vi "Disable.vi"(8 "error in (no error)":errorcluster, 11 "NHRDCPower in":refnum<class "NHRDCPower.lvclass">) -> (0 "error out":errorcluster, 3 "NHRDCPower out":refnum<class "NHRDCPower.lvclass">)   [LabVIEW 2018, in "AcPwrPlugins.lvlib" / "NHRDCPower.lvclass"]
doc: "This VI disconnects the instruments output or input."
uses:
  NHRDCPower.lvclass
  <instrlib>/NHRDCPowerModule/NHRDCPowerModule/NHRDCPowerModule.lvlib
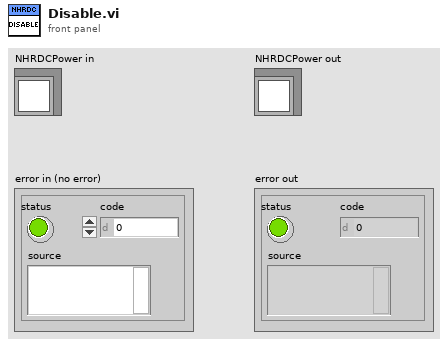
[diagram p1: front panel]
types:
  T1 = typedef "AcPwrPlugins.lvlib/NHRDCPower.lvclass/Device(s)Settings.ctl" = cluster{"Handle":string, "Name":string, "id query (Yes)":bool, "reset device (Yes)":bool, "Connected":bool, "Voltage Range (V)":dbl[], "Timing":cluster{"TimingOn":enum16{""}, "Hours":u32, "Minutes":u32, "Seconds":dbl, "CutoffVoltage":dbl}, "Initial Battery Detect Voltage (0)":sgl, "SafetySettings":cluster{"SetWatchDog":bool, "Voltage (V)":sgl, "Current (A)":sgl, "Power (W)":sgl, "Voltage Delay (s)":sgl, "Current Delay (s)":sgl, "Power Delay (s)":sgl}, "Options String":string, "Aperture Time (s)":sgl, "operating state (Off)":i32, "OutputSettings":cluster{"Voltage (V)":sgl, "Current (A)":sgl, "Resistance (Ohms)":sgl, "Power (W)":sgl, "Enable Voltage":bool, "Enable Current":bool, "Enable Resistance":bool, "Enable Power":bool, "Delay After (s)":sgl, "Wait Value (V, A, W)":sgl, "Enable Wait":bool, "Wait on Value":i32}[], "SlewRate":cluster{"Set Voltage Rate V/S":sgl, "Set Current Rate A/S":sgl, "Set Resistance Rate R/S":sgl, "Set Power Rate W/S":sgl}}[]
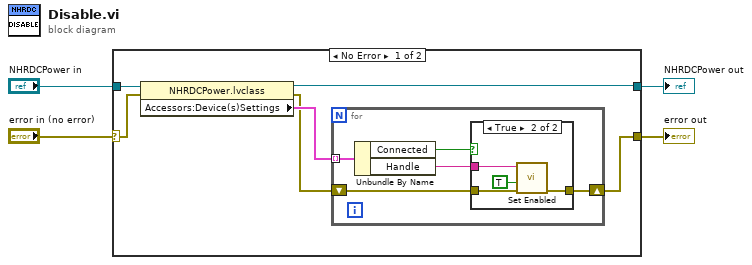
[diagram p0: block diagram]
diagram:
  n1 = case shown="No Error" "error in (no error)" {
    selector: "error in (no error)" -> [w9 w21]
    tunnel: [w5 w21] -> w1
    tunnel: [w6 w22] -> w2
    tunnel: "NHRDCPower in" -> [w10 w22]
    frame No Error {
      n2 = property class="NHRDCPower.lvclass"(reference=w10, error in=w9) -> (reference out=w6:refnum<class "NHRDCPower.lvclass">, error out=w7:errorcluster, "Accessors:Device(s)Settings"=w8:T1)
      n3 = for {
        tunnel: w8 -> [w15] mode=indexing
        shift-right: [w13] -> w5
        shift-left: w7 -> [w14]
        n4 = Unbundle By Name(w15) -> ("Connected"=w11:bool, "Handle"=w12:string)
        n5 = case shown="True" w11 {
          tunnel: w14 -> [w16 w19]
          tunnel: [w16 w20] -> w13
          tunnel: w12 -> [_ w18]
          frame False {
          }
          frame True {
            n6 = call <instrlib>:"Set Enabled.vi"("error in (no error)"=w19, "enabled (false)"=TRUE, "instrument handle"=w18) -> ("error out"=w20:errorcluster)  [unwired: 7 in, 1 out]
          }
        }
      }
    }
    frame Error {
    }
  }
  "error out" <- w1
  "NHRDCPower out" <- w2
